vi "Shooter Controller.vi"(8 "error in":errorcluster) -> ()   [LabVIEW 2016]
doc: "This VI executes continuously carrying out the current operation and responding to updates or new operations. It will often contain the timing or control code that is difficult to place directly in TeleOp. This VI generally opens all sensors and motors and isolates the rest of the robot code from knowing how the operations are carried out."
uses:
  Shooter Setpoints.ctl
  Shooter Operations.ctl
  <vilib>/Rock Robotics/WPI/ThirdParty/CanMotor/TalonSRX/WPI_CANTalonSRX_APIControlMode.ctl
  <vilib>/Rock Robotics/WPI/ThirdParty/CanMotor/TalonSRX/WPI_CANTalonSRX_APIFeedbackSelect.ctl
  <vilib>/Rock Robotics/SystemInterfaces/DIO/FPGA_DIOPWMChannel.ctl
panel:
  in  "Ramp Rate 2":dbl
  in  "F":dbl=0.09
  in  "D":dbl format="%#_13g"
  in  "I":dbl=-1000.0 format="%#_13g"
  in  "P":dbl=-0.04 format="%#_13g"
  out "Flywheel Speed":T1(graph)
  in  "F":dbl=0.012
  in  "D 2":dbl format="%#_13g"
  in  "I 2":dbl=3e-05 format="%#_13g"
  in  "P 2":dbl=0.017 format="%#_13g"
  in  "Edtit PID?":bool=TRUE
  out "Current\nCmd":string="Started at  Sat 15 Apr 2017 03:18:03 PM CDT\nDefault: Reserve,  S 0.0, D 0.000000"
  # "Tip: It may be helpful to observe inputs and sensor values.\nYou may also want to display tuning or debugging controls."
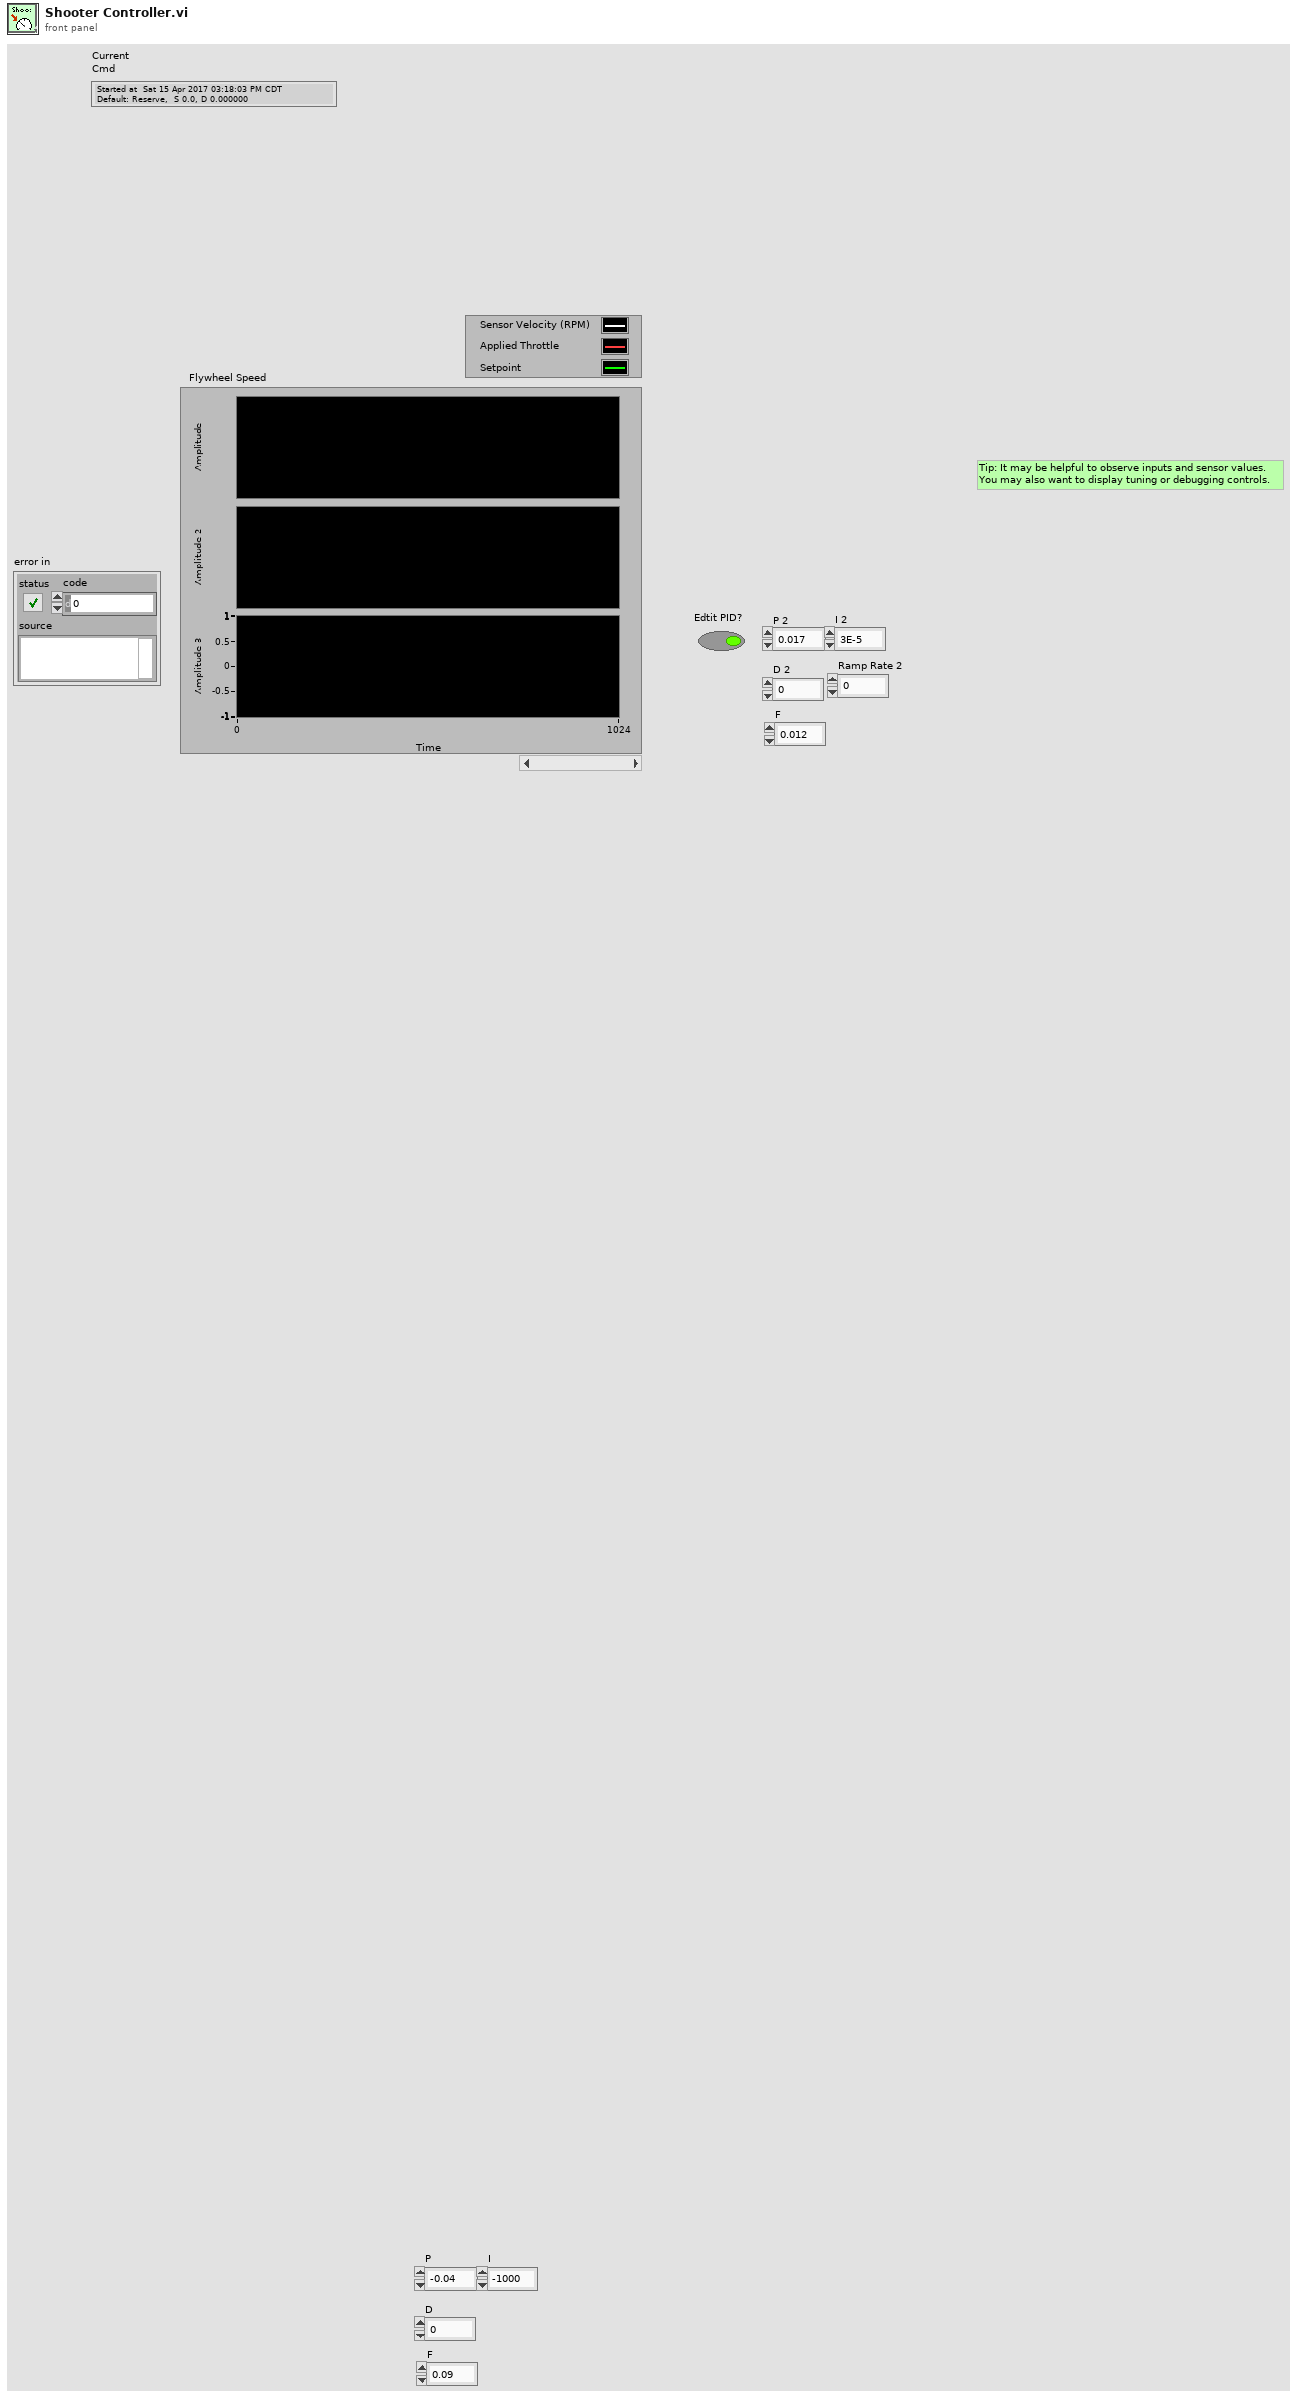
[diagram p1: front panel]
types:
  T1 = cluster{"Sensor Velocity":dbl, "Applied Throttle":dbl, "Output":dbl}
  T2 = typedef "FPGA_DIOPWMChannel.ctl" = enum8{"PWM 0", "PWM 1", "PWM 2", "PWM 3", "PWM 4", "PWM 5", "PWM 6", "PWM 7", "PWM 8", "PWM 9", "PWM MXP 0", "PWM MXP 1", "PWM MXP 2", "PWM MXP 3", "PWM MXP 4", "PWM MXP 5", "PWM MXP 6", "PWM MXP 7", "PWM MXP 8", "PWM MXP 9", "Invalid"}
  T3 = typedef "WPI_CANTalonSRX_APIFeedbackSelect.ctl" = enum16{"Digital Quadrature Encoder", "Analog Potentiometer", "Analog Encoder", "Count on Quad-A (Rising-Edge)", "Count on Quad-A (Falling-Edge)", "CTR Magnetic Enc (Absolute)", "CTR Magnetic Enc (Relative)", "Pulse Width"}
  T4 = typedef "WPI_CANTalonSRX_APIControlMode.ctl" = enum8{"Percent VBus", "Speed", "Position", "Slave", "Unchanged / Invalid", "Voltage Compensation", "Current", "Motion Profile", "Motion Magic"}
  T5 = typedef "Shooter Setpoints.ctl" = cluster{"Operation":T6, "Setpoint":dbl, "Hood Angle":dbl, "Speed (RPM)":dbl}
  T6 = typedef "Shooter Operations.ctl" = enum16{"Reserve", "Read Current", "Immediate", "Spin Flywheels", "Angle Hood", "Stop flywheels"}
  T7 = typedef "WPI_ServoDeviceRef.ctl" = cluster{"DeviceStatus":errorcluster, "PWM Channel":T2, "DeadBand":T8}
  T8 = typedef "WPI_PWMDeadband.ctl" = cluster{"Name":string, "maxPositivePwm":i32, "minPositivePwm":i32, "centerPwm":i32, "maxNegativePwm":i32, "minNegativePwm":i32, "angularRange":u16}
  T9 = typedef "WPI_MotorControlDeviceRef.ctl" = cluster{"DeviceStatus":errorcluster, "Type":T10, "PWM":cluster{"PWM Channel":T2, "DeadBand":T8}, "CAN":cluster{"Device Number":u8, "SetOutput VI Ref":variant, "GetOutput VI Ref":variant, "Enable VI Ref":variant, "Disable VI Ref":variant, "Data":variant}, "Invert":bool}
  T10 = typedef "WPI_MotorControlType.ctl" = enum16{"PWM", "CAN"}
  T11 = typedef "Command Status Info.ctl" = cluster{"Name":string, "Status":T12, "notifier out":T13}
  T12 = typedef "Completion Status.ctl" = enum16{"Successful", "Aborted", "Incomplete"}
  T13 = typedef "Completion Notifier.ctl" = refnum<notifier>
  T14 = cluster{"Default Command":T5, "Command Timing":cluster{"Start Time (ms)":u32, "Iterations":i32}, "Command Arguments":cluster{"Command Info":T11, "Description":string, "Default Command":T5, "notifier out":refnum<notifier>, "Subsystem Name":string}}
  T15 = typedef "WPI_CANTalonSRX_GlobalStatus.ctl" = cluster{"Applied Throttle":dbl, "Module Enabled":bool, "CAN Error":errorcluster, "Closed Loop Error":dbl, "Forward Limit Switch Closed":bool, "Reverse Limit Switch Closed":bool, "Sensor Position":dbl, "Sensor Velocity":dbl, "Current":dbl, "Sticky Fault - Over Temp":bool, "Sticky Fault - Under Voltage":bool, "Sticky Fault - Forward Limit":bool, "Sticky Fault - Reverse Limit":bool, "Sticky Fault - Forward Soft Limit":bool, "Sticky Fault - Reverse Soft Limit":bool, "Brake is Enabled":bool, "Encoder Position":dbl, "Encoder Velocity":dbl, "Encoder Index Count":dbl, "Encoder A Pin State":bool, "Encoder B Pin State":bool, "Encoder Index Pin State":bool, "Analog In":dbl, "Analog In Velocity":dbl, "Temperature (C)":dbl, "Battery Voltage":dbl, "Control 5 Is Supported":bool, "Current Profile Slot Select":dbl, "Pos Div 8":bool, "Vel Div 4":bool, "Pulse Width Position":i32, "Pulse Width Velocity":i32, "Pulse Width Rise To Rise (us)":i32, "Pulse Width Rise To Fall (us)":i32, "Mot Prof Active Is Under Run":bool, "Mot Prof Active Has Under Run":bool, "Mot Prof Active Is Last":bool, "Mot Prof Active Velocity Only":bool, "Mot Prof Active Is Valid":bool, "Mot Prof Buffer Is Full":bool, "Mot Prof Active Profile Slot Select":i32, "Mot Prof NextID":i32, "Mot Prof Count":i32, "Mot Prof Active Velocity":dbl, "Mot Prof Active Position":dbl, "Mot Prof Output Enable":i32, "UsageFrame":u32, "Motion Magic Active Trajectory":cluster{"Velocity":dbl, "Position":dbl}}
  T16 = cluster{dbl, "Applied Throttle":dbl, "Output":dbl}
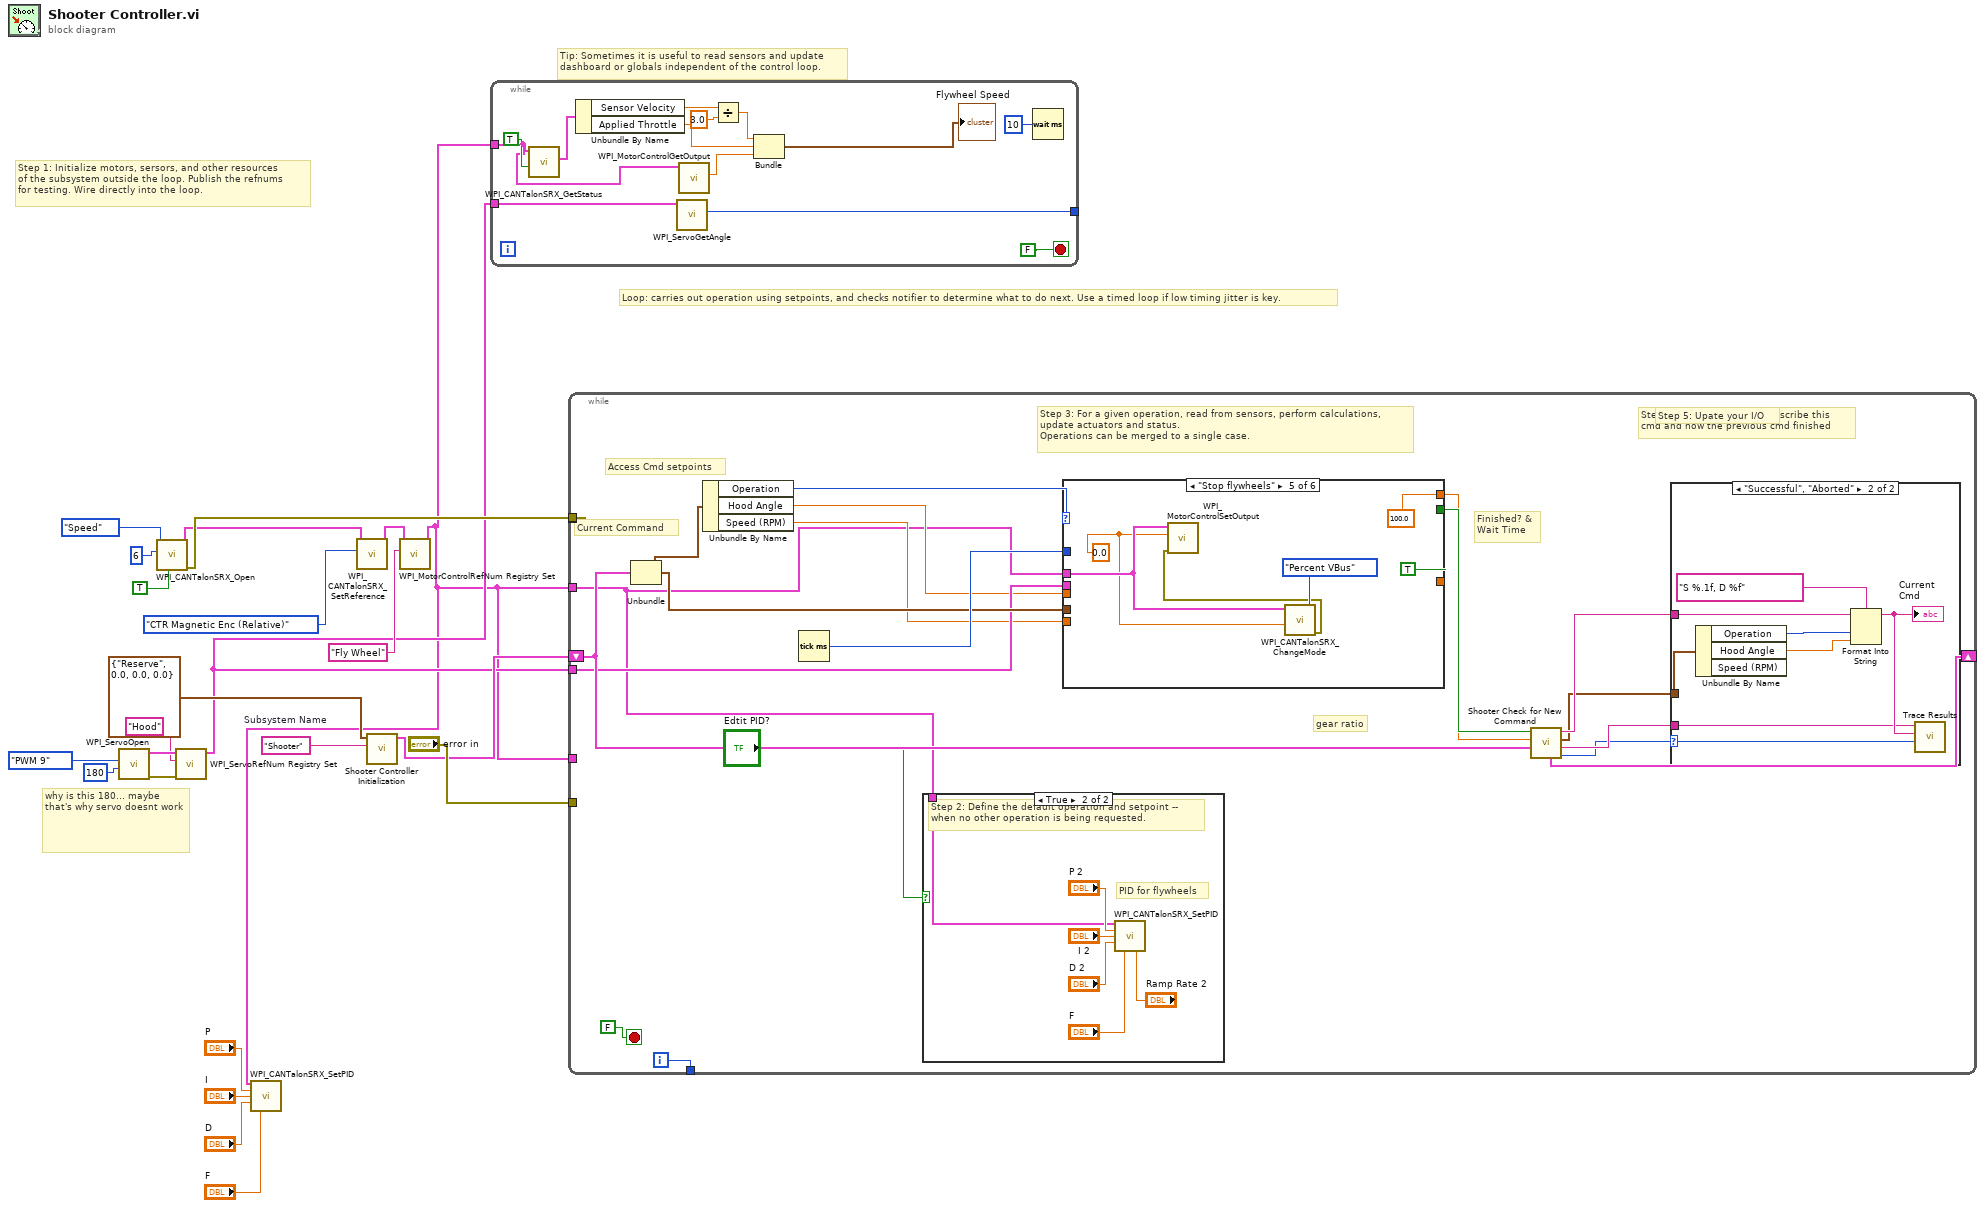
[diagram p0: block diagram]
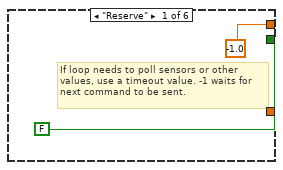
[diagram p2: hidden frame]
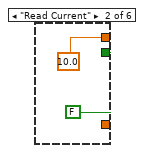
[diagram p3: hidden frame]
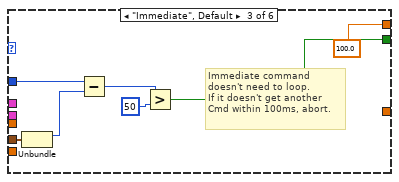
[diagram p4: hidden frame]
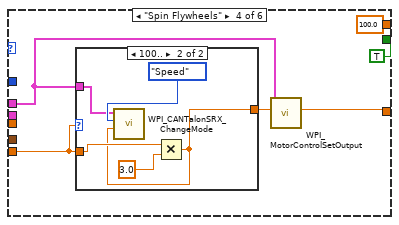
[diagram p5: hidden frame]
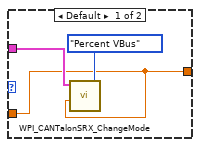
[diagram p6: hidden frame]
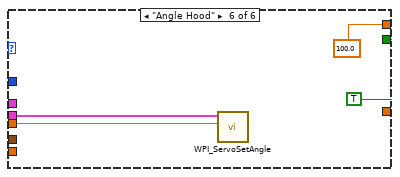
[diagram p7: hidden frame]
diagram:
  w22 = "Shooter"  # Subsystem Name
  # "why is this 180... maybe that's why servo doesnt work"
  # "Tip: Sometimes it is useful to read sensors and update\ndashboard or globals independent of the control loop."
  # "Step 1: Initialize motors, sersors, and other resources\nof the subsystem outside the loop. Publish the refnums\nfor testing. Wire directly into the loop."
  # "Loop: carries out operation using setpoints, and checks notifier to determine what to do next. Use a timed loop if low timing jitter is key."
  n1 = call <vilib>:"WPI_ServoOpen.vi"("Angular Range"=u16 180, "PWM Channel"=FPGA_DIOPWMChannel."PWM 9") -> ("error out"=w9:errorcluster, "ServoDeviceRef"=w13:T7)  [unwired: 8 in]
  n2 = call <vilib>:"WPI_CANTalonSRX_Open.vi"("Invert"=TRUE, "Device Number"=u8 6, "Control Mode"=WPI_CANTalonSRX_APIControlMode."Speed") -> ("error out"=w17:errorcluster, "CAN Talon SRX Ref"=w16:T9)  [unwired: 7 in]
  n3 = call <vilib>:"WPI_ServoRefNum Registry Set.vi"("error in (no error)"=w9, "refnum name"="Hood", "ServoDeviceRef"=w13) -> ("ServoDeviceRef"=w8:T7)  [unwired: 7 in, 1 out]
  n4 = call <vilib>:"WPI_CANTalonSRX_SetReference.vi"("Feedback Reference"=WPI_CANTalonSRX_APIFeedbackSelect."CTR Magnetic Enc (Relative)", "CAN Talon SRX Ref"=w16) -> ("CAN Talon SRX Ref"=w15:T9)  [unwired: 8 in, 1 out]
  n5 = call "Shooter Controller Initialization.vi"("Subsystem Name"=w22, "Default Command"=T5 {"Operation"=enum."Reserve", "Setpoint"=0.0, "Hood Angle"=0.0, "Speed (RPM)"=0.0} ("SubSystem Data")) -> ("Command Info"=w20:T14)  [unwired: 9 in]
  n6 = call <vilib>:"WPI_MotorControlRefNum Registry Set.vi"("refnum name"="Fly Wheel", "MotorControlDevRef"=w15) -> ("MotorControlDevRef"=w2:T9)  [unwired: 8 in, 1 out]
  n7 = call <vilib>:"WPI_CANTalonSRX_SetPID.vi"("CAN Talon SRX Ref"=w2, "P"="P", "I"="I", "D"="D", "F"="F") -> ()  [unwired: 9 in, 2 out]
  n8 = while {
    tunnel: w2 -> [w27]
    tunnel: w8 -> [w32]
    tunnel: [w31] -> _
    stop <- FALSE stop-if-true
    n9 = call <vilib>:"WPI_CANTalonSRX_GetStatus.vi"("Clear Sticky Faults"=TRUE, "CAN Talon SRX Ref"=w27) -> ("Talon SRX Status"=w33:T15)  [unwired: 7 in, 2 out]
    n10 = Unbundle By Name(w33) -> ("Sensor Velocity"=w25:dbl, "Applied Throttle"=w30:dbl)
    n11 = call <vilib>:"WPI_ServoGetAngle.vi"("ServoDeviceRef"=w32) -> ("Angle"=w31:u16)  [unwired: 7 in, 2 out]
    n12 = call <vilib>:"WPI_MotorControlGetOutput.vi"("MotorControlDevRef"=w27) -> ("Output"=w28:dbl)  [unwired: 8 in, 2 out]
    n13 = Divide(x=w25, y=3.0 ("x")) -> (x/y=w24:dbl)
    n14 = Bundle(w24, "Applied Throttle"=w30, "Output"=w28) -> (→"Flywheel Speed":T16)  [unwired: 1 in]
    n15 = Wait (ms)(milliseconds to wait=u32 10) -> ()  [unwired: 1 out]
  }
  n16 = while {
    tunnel: [w55] -> _
    tunnel: "error in" -> [_]
    tunnel: w2 -> [w37]
    shift-right: [w43] -> _
    shift-left: w20 -> [w44]
    tunnel: w8 -> [w42]
    tunnel: w2 -> [_]
    tunnel: [w39] -> _
    tunnel: w17 -> [w39]
    i -> [w55]
    stop <- FALSE stop-if-true
    # "gear ratio"
    # "Step 5: Upate your I/O"
    # "Step 4: Format a string to describe this\ncmd and how the previous cmd finished"
    # "Current Command"
    # "Access Cmd setpoints"
    # "Finished? &\nWait Time"
    # "Step 3: For a given operation, read from sensors, perform calculations,\nupdate actuators and status.\nOperations can be merged to a single case."
    n17 = Unbundle(w44) -> ("Default Command"=w54:T5, "Command Timing"=w51:cluster{"Start Time (ms)":u32, "Iterations":i32})  [unwired: 1 out]
    n18 = Unbundle By Name(w54) -> ("Operation"=w53:T6, "Hood Angle"=w41:dbl, "Speed (RPM)"=w40:dbl)
    n19 = Tick Count (ms)() -> (millisecond timer value=w52:u32)
    n20 = case shown="True" "Edtit PID?" {
      tunnel: w37 -> [_ w102]
      frame False {
      }
      frame True {
        # "PID for flywheels"
        # "Step 2: Define the default operation and setpoint --\nwhen no other operation is being requested."
        n21 = call <vilib>:"WPI_CANTalonSRX_SetPID.vi"("CAN Talon SRX Ref"=w102, "P"="P 2", "I"="I 2", "D"="D 2", "F"="F", "Ramp Rate"="Ramp Rate 2") -> ()  [unwired: 8 in, 2 out]
      }
    }
    n22 = case shown="\"Stop flywheels\"" w53 {
      tunnel: [-1.0 10.0 100.0 100.0 100.0 100.0] -> w49
      tunnel: [FALSE ("ignore previous (F)") FALSE ("ignore previous (F)") w61 TRUE ("ignore previous (F)") TRUE ("ignore previous (F)") TRUE ("ignore previous (F)")] -> w50
      tunnel: w51 -> [_ _ w63 _ _ _]
      tunnel: w52 -> [_ _ w62 _ _ _]
      tunnel: w37 -> [_ _ _ w69 w84 _]
      tunnel: w42 -> [_ _ _ _ _ w91]
      tunnel: w41 -> [_ _ _ _ _ w88]
      tunnel: w40 -> [_ _ _ w68 _ _]
      tunnel: [_ _ _ w70 _ _] -> _
      frame "Reserve" {
        # "If loop needs to poll sensors or other\nvalues, use a timeout value. -1 waits for\nnext command to be sent."
      }
      frame "Read Current" {
      }
      frame "Immediate", Default {
        # "Immediate command\ndoesn't need to loop.\nIf it doesn't get another\nCmd within 100ms, abort."
        n23 = Unbundle(w63) -> ("Start Time (ms)"=w66:u32)  [unwired: 1 out]
        n24 = Subtract(x=w62, y=w66) -> (x-y=w65:u32)
        n25 = Greater?(x=w65, y=u8 50 ("Left Motor")) -> (0:w61:bool)
      }
      frame "Spin Flywheels" {
        n26 = case shown="100.." w68 {
          tunnel: [w74 w77] -> w71
          tunnel: w68 -> [w74 w81]
          tunnel: w69 -> [w76 w78]
          frame Default {
            n27 = call <vilib>:"WPI_CANTalonSRX_ChangeMode.vi"("Output"=w74, "Control Mode"=WPI_CANTalonSRX_APIControlMode."Percent VBus", "CAN Talon SRX Ref"=w76) -> ()  [unwired: 7 in, 2 out]
          }
          frame 100.. {
            n28 = Multiply(x=w81, y=3.0) -> (x*y=w77:dbl)
            n29 = call <vilib>:"WPI_CANTalonSRX_ChangeMode.vi"("Output"=w77, "Control Mode"=WPI_CANTalonSRX_APIControlMode."Speed", "CAN Talon SRX Ref"=w78) -> ()  [unwired: 7 in, 2 out]
          }
        }
        n30 = call <vilib>:"WPI_MotorControlSetOutput.vi"("Output"=w71, "MotorControlDevRef"=w69) -> ("Motor Output"=w70:dbl)  [unwired: 7 in, 2 out]
      }
      frame "Stop flywheels" {
        w82 = 0.0 ("Output")
        n31 = call <vilib>:"WPI_CANTalonSRX_ChangeMode.vi"("Output"=w82, "Control Mode"=WPI_CANTalonSRX_APIControlMode."Percent VBus", "CAN Talon SRX Ref"=w84) -> ("error out"=w83:errorcluster)  [unwired: 7 in, 1 out]
        n32 = call <vilib>:"WPI_MotorControlSetOutput.vi"("error in (no error)"=w83, "Output"=w82, "MotorControlDevRef"=w84) -> ()  [unwired: 6 in, 3 out]
      }
      frame "Angle Hood" {
        n33 = call <vilib>:"WPI_ServoSetAngle.vi"("Angle"=w88, "ServoDeviceRef"=w91) -> ()  [unwired: 8 in, 2 out]
      }
    }
    n34 = call "Shooter Check for New Command.vi"("Current Command"=w44, "Wait time (ms)"=w49, "Finished?"=w50) -> ("Completion"=w45:T12, "Subsystem Name"=w46:string, "Current Command"=w47:T5, "Initial Trace String"=w48:string, "NextCommand"=w43:T14)  [unwired: 4 in]
    n35 = case shown="\"Successful\", \"Aborted\"" w45 {
      selector: w45 -> [_ w99]
      tunnel: w48 -> [_ w95]
      tunnel: w47 -> [_ w96]
      tunnel: w46 -> [_ w92]
      frame "Incomplete", Default {
        # "Continuing current command"
      }
      frame "Successful", "Aborted" {
        # "Report and setup for next command"
        n36 = Unbundle By Name(w96) -> ("Operation"=w98:T6, "Hood Angle"=w93:dbl)  [unwired: 1 out]
        n37 = Format Into String(format string="S %.1f, D %f", initial string=w95, w98, w93) -> (resulting string=w94:string)  [unwired: 1 in, 1 out]
        "Current\nCmd" <- w94
        n38 = call <vilib>:"Trace Results.vi"("Status of previous command"=w99, "Description"=w94, "Subsystem"=w92) -> ()  [unwired: 9 in]
      }
    }
  }
